vi "Get 8-bit PixMap.vi"(10 "Original Bit depth":i32, 11 "Color Data":u16[][][](array[numeric])) -> (3 "new picture":picture)   [LabVIEW 2020]
uses:
  <vilib>/picture/picture.llb/Draw True-Color Pixmap.vi
panel:
  out "Intensity Graph":u32[][](graph)
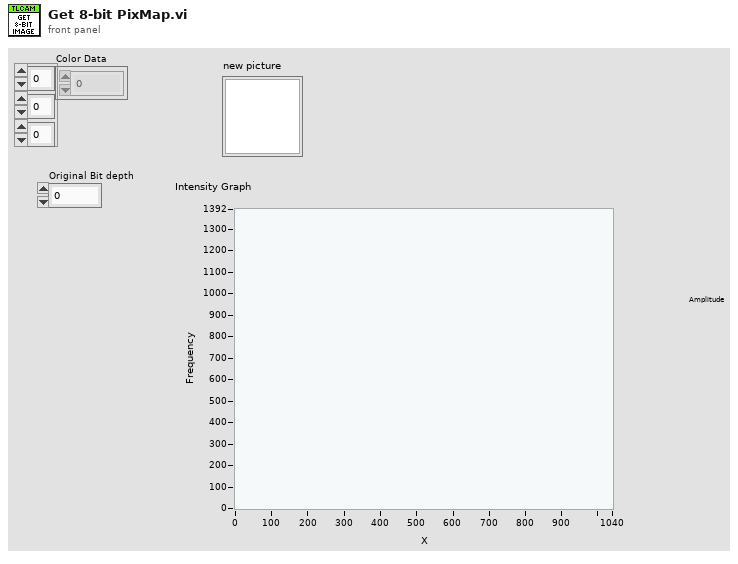
[diagram p1: front panel]
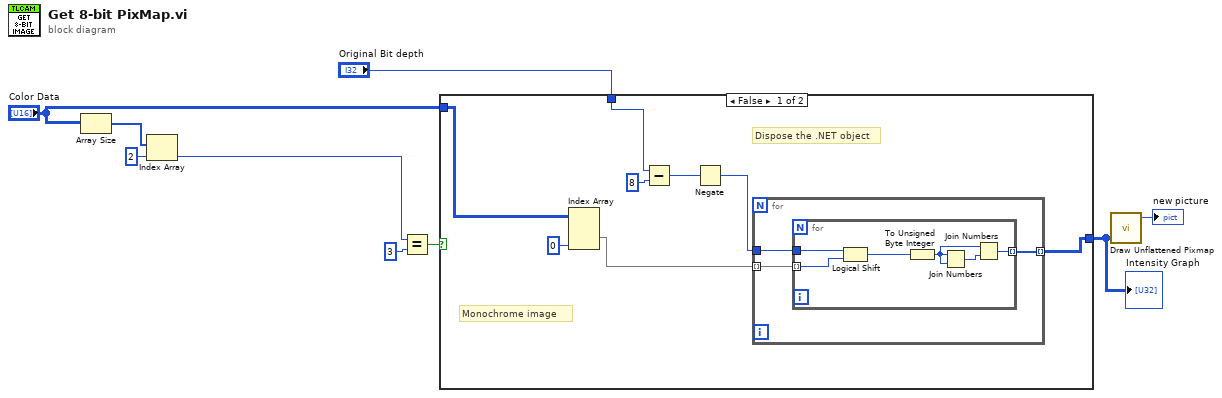
[diagram p0: block diagram]
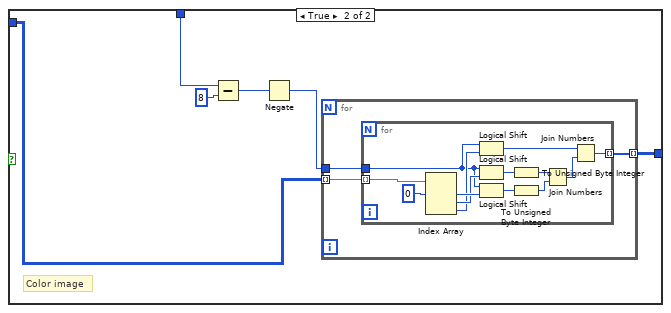
[diagram p2: hidden frame]
diagram:
  n1 = Array Size(array="Color Data") -> (size(s)=w6:i32[])
  n2 = Index Array(array=w6, index=2) -> (element=w2:i32)
  n3 = Equal?(x=w2, y=3) -> (x = y?=w7:bool)
  n4 = case shown="False" w7 {
    tunnel: [w14 w29] -> w1
    tunnel: "Color Data" -> [w12 w28]
    tunnel: "Original Bit depth" -> [w13 w27]
    frame False {
      # "Dispose the .NET object"
      # "Monochrome image"
      n5 = Index Array(array=w12, index (dim 2)=0 ("disabled index (col)")) -> (element=w10:u16[][])  [unwired: 2 in]
      n6 = Subtract(x=w13, y=8) -> (x-y=w16:i32)
      n7 = Negate(x=w16) -> (-x=w15:i32)
      n8 = for {
        tunnel: w10 -> [w20] mode=indexing
        tunnel: w15 -> [w19]
        tunnel: [w18] -> w14 mode=indexing
        n9 = for {
          tunnel: w20 -> [w22] mode=indexing
          tunnel: w19 -> [w26]
          tunnel: [w23] -> w18 mode=indexing
          n10 = Logical Shift(y=w26, x=w22) -> (x << y=w24:u16)
          n11 = To Unsigned Byte Integer(number=w24) -> (unsigned 8bit integer=w21:u8)
          n12 = Join Numbers(hi=w21, lo=w21) -> ((hi.lo)=w25:u16)
          n13 = Join Numbers(hi=w21, lo=w25) -> ((hi.lo)=w23:u32)
        }
      }
    }
    frame True {
      # "Color image"
      n14 = Subtract(x=w27, y=8) -> (x-y=w31:i32)
      n15 = Negate(x=w31) -> (-x=w30:i32)
      n16 = for {
        tunnel: w28 -> [w35] mode=indexing
        tunnel: w30 -> [w34]
        tunnel: [w33] -> w29 mode=indexing
        n17 = for {
          tunnel: w35 -> [w48] mode=indexing
          tunnel: w34 -> [w43]
          tunnel: [w37] -> w33 mode=indexing
          n18 = Index Array(array=w48, index #1=0 ("index")) -> (element #1=w46:u16, element #2=w45:u16, element #3=w44:u16)  [unwired: 2 in]
          n19 = Logical Shift(y=w43, x=w44) -> (x << y=w36:u16)
          n20 = Logical Shift(y=w43, x=w45) -> (x << y=w40:u16)
          n21 = Logical Shift(y=w43, x=w46) -> (x << y=w41:u16)
          n22 = To Unsigned Byte Integer(number=w40) -> (unsigned 8bit integer=w38:u8)
          n23 = To Unsigned Byte Integer(number=w41) -> (unsigned 8bit integer=w39:u8)
          n24 = Join Numbers(hi=w38, lo=w39) -> ((hi.lo)=w42:u16)
          n25 = Join Numbers(hi=w36, lo=w42) -> ((hi.lo)=w37:u32)
        }
      }
    }
  }
  "Intensity Graph" <- w1
  n26 = call-poly <vilib>:"Draw Unflattened Pixmap.vi"("data (RGB format)"=w1) -> ("new picture"=→"new picture":picture)  [unwired: 8 in]
